vi "Find and trigger default events.vi"(9 "Event to Trigger":string, 10 "Library Selected":string, 11 "References Map":map{string, refnum<vi>}(c390)) -> (0 "error out":errorcluster)   [LabVIEW 2020, in "Panther Dashboard.lvlib"]
uses:
  Panther Dashboard.lvlib
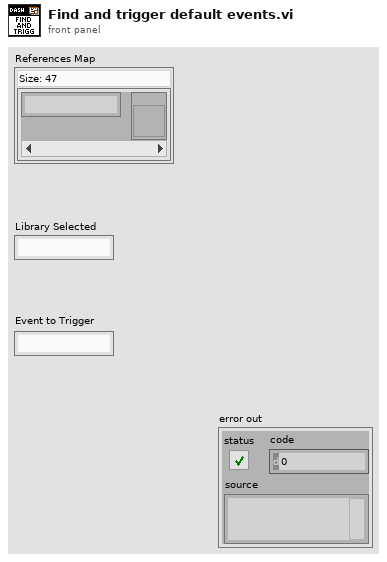
[diagram p1: front panel]
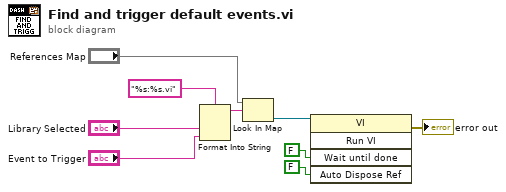
[diagram p0: block diagram]
diagram:
  n1 = Format Into String(format string="%s:%s.vi", "Library Selected", "Event to Trigger") -> (resulting string=w2:string)  [unwired: 2 in, 1 out]
  n2 = Look In Map(map="References Map", key=w2) -> (value=w6:refnum<vi>)  [unwired: 1 in, 1 out]
  n3 = invoke class="VI" method="Run VI"(reference=w6, "Wait until done"=FALSE ("Wait Until Done"), "Auto Dispose Ref"=FALSE ("Auto Dispose Reference")) -> (error out=→"error out":errorcluster)  [unwired: 2 in, 4 out]
